vi "Set RPC PerformOCVMeasurement __Output.vi"(7 "Streeming? (F)":bool, 8 "error in (no error)":errorcluster, 10 "Message Data":T1, 11 "gRPCid in":T4) -> (0 "error out":errorcluster)   [LabVIEW 2019, in "OCV2.lvlib" / "OCV2.lvclass"]
uses:
  OCV2.lvclass
  gRPC lvSupport/Server API/typeDefs/grpcId.ctl
  RPC Messages/measurementservice_OCVData/measurementservice_OCVData_Data.ctl
  RPC Messages/measurementservice_OCVRaw/measurementservice_OCVRaw_Data.ctl
  RPC Messages/measurementservice_ErrorOut/measurementservice_ErrorOut_Data.ctl
  gRPC lvSupport/gprc-lvsupport.lvlib
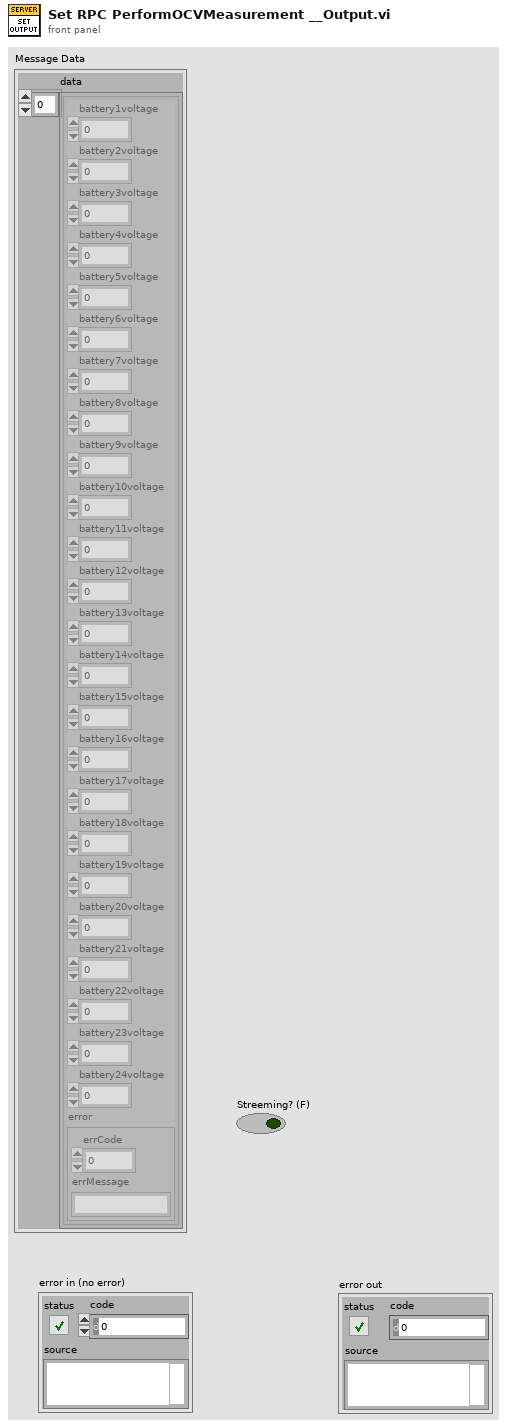
[diagram p1: front panel]
types:
  T1 = typedef "OCV2.lvlib/OCV2.lvclass/measurementservice_OCVData_Data.ctl" = cluster{"data":T2[]}
  T2 = typedef "OCV2.lvlib/OCV2.lvclass/measurementservice_OCVRaw_Data.ctl" = cluster{"battery1voltage":sgl, "battery2voltage":sgl, "battery3voltage":sgl, "battery4voltage":sgl, "battery5voltage":sgl, "battery6voltage":sgl, "battery7voltage":sgl, "battery8voltage":sgl, "battery9voltage":sgl, "battery10voltage":sgl, "battery11voltage":sgl, "battery12voltage":sgl, "battery13voltage":sgl, "battery14voltage":sgl, "battery15voltage":sgl, "battery16voltage":sgl, "battery17voltage":sgl, "battery18voltage":sgl, "battery19voltage":sgl, "battery20voltage":sgl, "battery21voltage":sgl, "battery22voltage":sgl, "battery23voltage":sgl, "battery24voltage":sgl, "error":T3}
  T3 = typedef "OCV2.lvlib/OCV2.lvclass/measurementservice_ErrorOut_Data.ctl" = cluster{"errCode":i32, "errMessage":string}
  T4 = typedef "OCV2.lvlib/gprc-lvsupport.lvlib/grpcId.ctl" = u64
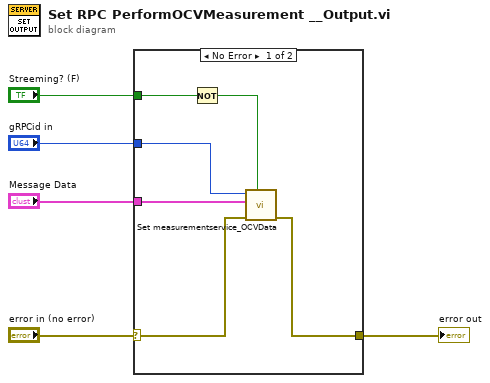
[diagram p0: block diagram]
diagram:
  n1 = case shown="No Error" "error in (no error)" {
    selector: "error in (no error)" -> [w11 w12]
    tunnel: [w9 w12] -> w4
    tunnel: "gRPCid in" -> [w10 _]
    tunnel: "Message Data" -> [w8 _]
    tunnel: "Streeming? (F)" -> [w7 _]
    frame No Error {
      n2 = Not(x=w7) -> (.not. x?=w6:bool)
      n3 = call "Set measurementservice_OCVData.vi"("Complete Call (T)"=w6, "error in (no error)"=w11, "Message Data"=w8, "gRPCid"=w10) -> ("error out"=w9:errorcluster)  [unwired: 7 in]
    }
    frame Error {
    }
  }
  "error out" <- w4
